vi "Sensor to Certainty graph.vi"(6 "Distance":fxp<+/-,64,32>, 8 "Degrees":dbl, 9 "Sensor y":i16, 10 "Sensor x":i16, 11 "Array 2":i16[][](array[numeric])) -> (3 "Array 3":i16[][](array[numeric]))   [LabVIEW 2012]
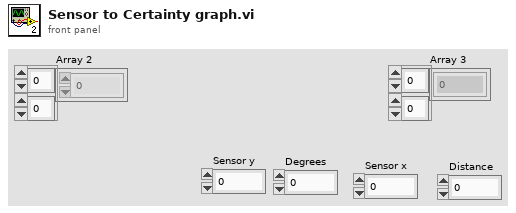
[diagram p1: front panel]
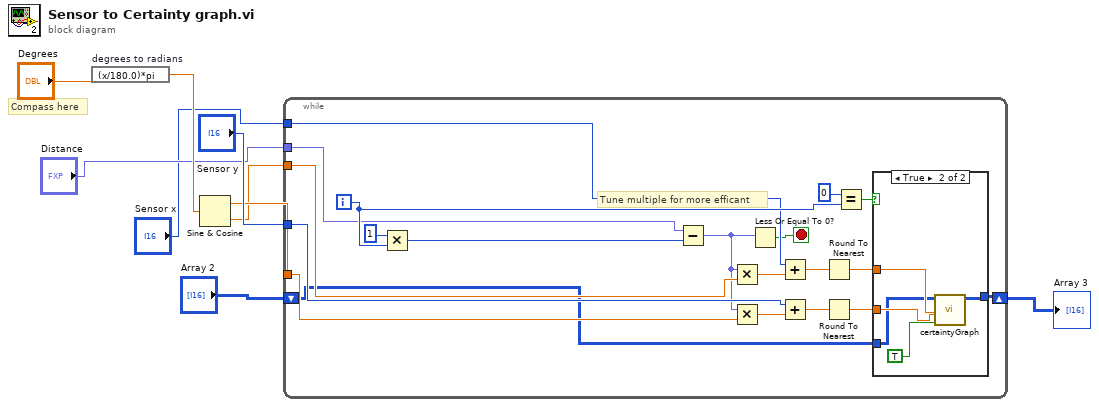
[diagram p0: block diagram]
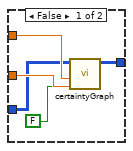
[diagram p2: hidden frame]
diagram:
  # "Compass here"
  n1 = expression code="(x/180.0)*pi" "degrees to radians"("Degrees") -> (w7:dbl)
  n2 = Sine & Cosine(0:w7) -> (1:w6:dbl, 2:w5:dbl)
  n3 = while {
    tunnel: "Sensor y" -> [w15]
    tunnel: "Sensor x" -> [w14]
    tunnel: "Distance" -> [w22]
    tunnel: w6 -> [w20]
    tunnel: w5 -> [w21]
    shift-right: [w10] -> w1
    shift-left: "Array 2" -> [w13]
    i -> [w25]
    stop <- w11 stop-if-true
    # "Tune multiple for more efficant"
    n4 = Multiply(x=1, y=w25) -> (x*y=w23:i32)
    n5 = Subtract(x=w22, y=w23) -> (x-y=w12:fxp<+/-,64,33>)
    n6 = Multiply(x=w12, y=w21) -> (x*y=w19:dbl)
    n7 = Multiply(x=w12, y=w20) -> (x*y=w18:dbl)
    n8 = Less Or Equal To 0?(x=w12) -> (x <= 0?=w11:bool)
    n9 = Add(x=w14, y=w19) -> (x+y=w17:dbl)
    n10 = Add(x=w15, y=w18) -> (x+y=w16:dbl)
    n11 = Round To Nearest(number=w17) -> (nearest integer value=w26:dbl)
    n12 = Round To Nearest(number=w16) -> (nearest integer value=w27:dbl)
    n13 = Equal?(x=0, y=w25) -> (x = y?=w28:bool)
    n14 = case shown="True" w28 {
      tunnel: w26 -> [w34 w38]
      tunnel: w27 -> [w33 w37]
      tunnel: w13 -> [w31 w36]
      tunnel: [w30 w35] -> w10
      frame False {
        n15 = call "certaintyGraph.vi"("Detected"=FALSE, "Y"=w33, "X"=w34, "Array"=w31) -> ("Array 2"=w30:i16[][])  [unwired: 7 in]
      }
      frame True {
        n16 = call "certaintyGraph.vi"("Detected"=TRUE, "Y"=w37, "X"=w38, "Array"=w36) -> ("Array 2"=w35:i16[][])  [unwired: 7 in]
      }
    }
  }
  "Array 3" <- w1
